vi "SetList Columns to Devices.vi"(8 "error in (no error)":errorcluster, 9 "Col array in":refnum<class "Column.lvclass">[](array[class]), 10 "DevNums In":i32[](array[numeric]), 11 "Devices queue":refnum<queue>) -> (0 "error out":errorcluster, 3 "Devices queue out":refnum<queue>)   [LabVIEW 2013]
doc: "Loop over devices and set corresponding columns from Table's column array. (Appearance only, not SWI data!)\nThis VI is read-only w.r.t column data."
uses:
  ColumnVIs/Column/Column.lvclass
  Device/Device.lvclass
panel:
  # "Want to update SetList Appearance changes to devices!"
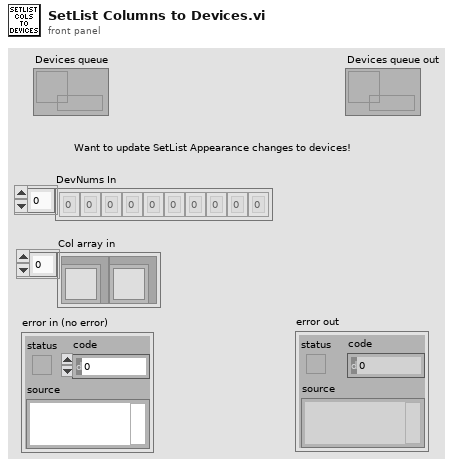
[diagram p1: front panel]
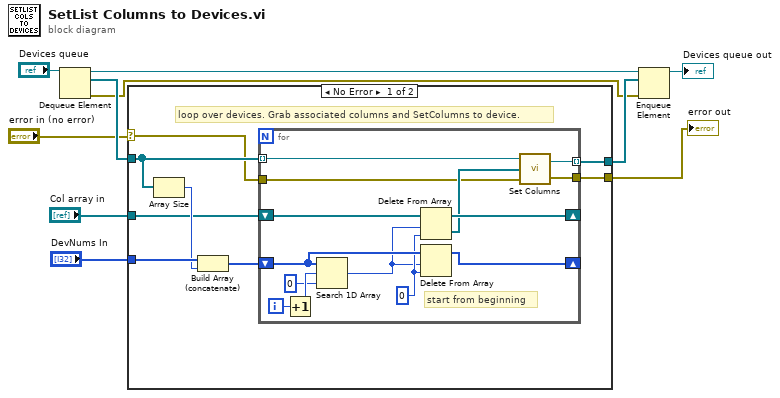
[diagram p0: block diagram]
diagram:
  n1 = Dequeue Element(queue="Devices queue") -> (queue out=w6:refnum<queue>, element=w7:refnum<class "Device.lvclass">[], error out=w1:errorcluster)  [unwired: 2 in, 1 out]
  n2 = case shown="No Error" "error in (no error)" {
    selector: "error in (no error)" -> [w11 w34]
    tunnel: [w18 w33] -> w5
    tunnel: w7 -> [w17 w33]
    tunnel: "DevNums In" -> [w16 _]
    tunnel: "Col array in" -> [w13 _]
    tunnel: [w12 w34] -> w2
    frame No Error {
      # "loop over devices. Grab associated columns and SetColumns to device."
      n3 = Array Size(array=w17) -> (size(s)=w14:i32)
      n4 = Build Array (concatenate)(w16, w14) -> (w15:i32[])
      n5 = for {
        tunnel: w17 -> [w32] mode=indexing
        tunnel: [w31] -> w18 mode=indexing
        shift-right: [w27] -> _
        shift-left: w13 -> [w28]
        shift-right: [w24] -> _
        shift-left: w15 -> [w25]
        tunnel: [w20] -> w12
        tunnel: w11 -> [w19]
        i -> [w30]
        w22 = 0 ("start index (0)")
        # "start from beginning"
        n6 = Increment(x=w30) -> (x+1=w29:i32)
        n7 = Search 1D Array(1D array=w25, element=w29, start index (0)=0) -> (index of element=w21:i32)
        n8 = Delete From Array(array=w28, length=w21, index=w22) -> (deleted portion=w26:refnum<class "Column.lvclass">[], array with subset deleted=w27:refnum<class "Column.lvclass">[])
        n9 = Delete From Array(array=w25, length=w21, index=w22) -> (array with subset deleted=w24:i32[])  [unwired: 1 out]
        n10 = call-dynamic "Set Columns.vi"("error in (no error)"=w19, "Columns"=w26, "Device in"=w32) -> ("error out"=w20:errorcluster, "Device out"=w31:refnum<class "Device.lvclass">)  [unwired: 1 in]
      }
    }
    frame Error {
    }
  }
  "error out" <- w2
  n11 = Enqueue Element(queue=w6, element=w5, error in (no error)=w1) -> (queue out=→"Devices queue out":refnum<queue>)  [unwired: 1 in, 2 out]
